vi "FilterSignalList.vi"(8 "Error in":errorcluster, 10 "SignalTypeToFilter":i32(ring)=1 items=["Measurable"=1, "AnalogIn"=2, "AnalogOut"=4, "DigitalIn"=8, "DigitalOut"=16, "Virtual"=32], 11 "DevicesAndSignals":T1) -> (0 "Error out":errorcluster, 3 "DevicesAndSignals":T1)   [LabVIEW 2016]
doc: "Filters all given signals according to the given signal type.\n\nSignalTypeToFilter: Signal type (you may add different signal types, e.g.: DigitalOut + AnalogOut) you want to filter. After execution the devices and signals output contains these signals only."
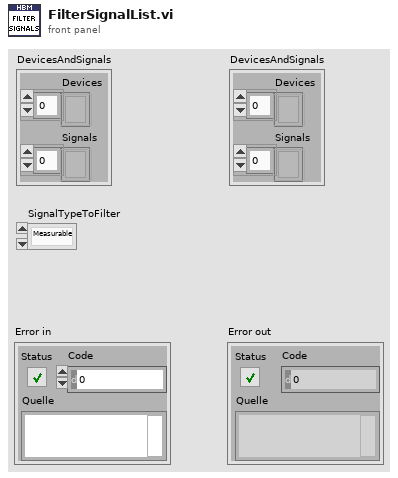
[diagram p1: front panel]
types:
  T1 = cluster{"Devices":refnum<k24>[], "Signals":refnum<k24>[]}
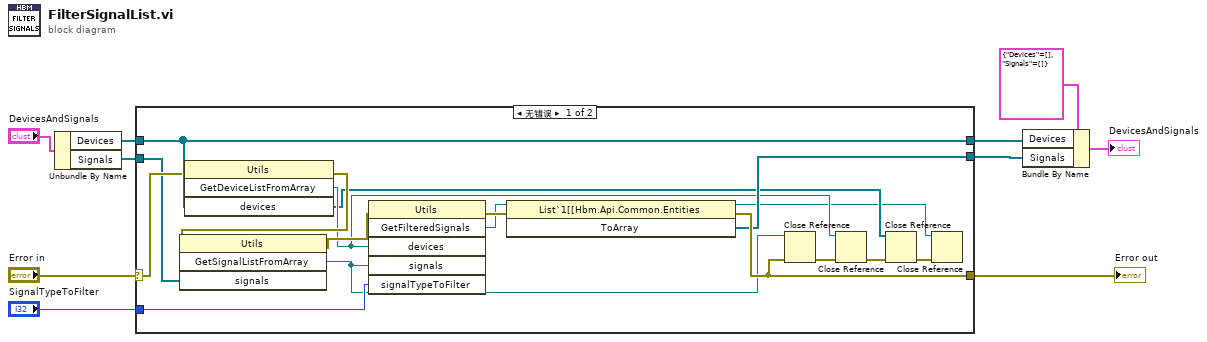
[diagram p0: block diagram]
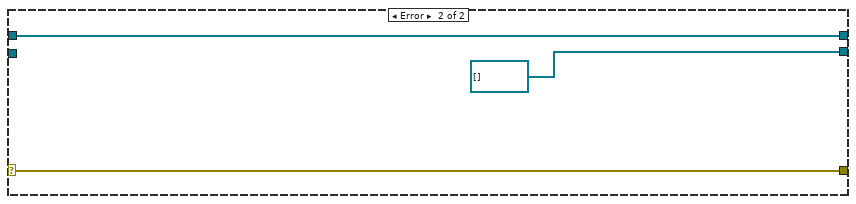
[diagram p2: hidden frame]
diagram:
  n1 = Unbundle By Name("DevicesAndSignals") -> ("Devices"=w3:refnum<k24>[], "Signals"=w2:refnum<k24>[])
  n2 = case shown="无错误" "Error in" {
    selector: "Error in" -> [w24 w30]
    tunnel: [w20 w30] -> w10
    tunnel: [w19 refnum<k24>[] [] ("ToArray")] -> w5
    tunnel: w3 -> [w27 w28]
    tunnel: [w27 w28] -> w6
    tunnel: w2 -> [w12 _]
    tunnel: "SignalTypeToFilter" -> [w21 _]
    frame No Error {
      n3 = invoke on="Methodenknoten" class="Utils" method="GetDeviceListFromArray"(error in=w24, "devices"=w27) -> (error out=w23:errorcluster, "GetDeviceListFromArray"=w16:refnum<k24>, "devices"=w14:refnum<k24>[])  [unwired: 2 in, 1 out]
      n4 = invoke on="Methodenknoten" class="Utils" method="GetSignalListFromArray"(error in=w23, "signals"=w12) -> (error out=w22:errorcluster, "GetSignalListFromArray"=w18:refnum<k24>)  [unwired: 2 in, 2 out]
      n5 = invoke on="Methodenknoten" class="Utils" method="GetFilteredSignals"(error in=w22, "devices"=w16, "signals"=w18, "signalTypeToFilter"=w21) -> (error out=w26:errorcluster, "GetFilteredSignals"=w25:refnum<k24>)  [unwired: 2 in, 4 out]
      n6 = invoke on="Methodenknoten" class="List`1[[Hbm.Api.Common.Entities" method="ToArray"(reference=w25, error in=w26) -> (reference out=w11:refnum<k24>, error out=w20:errorcluster, "ToArray"=w19:refnum<k24>[])  [unwired: 1 in]
      n7 = Close Reference(reference=w18, error in (no error)=w20) -> (error out=w17:errorcluster)
      n8 = Close Reference(reference=w16, error in (no error)=w17) -> (error out=w15:errorcluster)
      n9 = Close Reference(reference=w14, error in (no error)=w15) -> (error out=w13:errorcluster)
      n10 = Close Reference(reference=w11, error in (no error)=w13) -> ()  [unwired: 1 out]
    }
    frame Error {
    }
  }
  "Error out" <- w10
  n11 = Bundle By Name(cluster=T1 {"Devices"=[], "Signals"=[]} ("DevicesAndSignals"), "Devices"=w6, "Signals"=w5) -> (→"DevicesAndSignals":T1)
